vi "Get En and Ref Channels.vi"(11 "Reply Payload":T1 {"Settings"."EEG Channels"."16 EEG Channels"."Channel No" step=1}) -> (1 "Ch Names":string[](array[string]), 2 "Referenced Channels":u16, 3 "Enabled Channels":u16)   [LabVIEW 2016, in "Lab Streaming Layer.lvlib"]
uses:
  Lab Streaming Layer.lvlib
  Settings Editor/Update Application Settings (Reply Payload)--cluster.ctl
  Settings Editor/Settings--cluster.ctl
  Acquisition/Signal Type--enum.ctl
  Acquisition/Calibration Values--cluster.ctl
  CML Shared/EEG Channel Settings.ctl
  Acquisition/Acquisition.lvlib
  CML Shared/CML Shared.lvlib
  Settings Editor/Settings Editor.lvlib
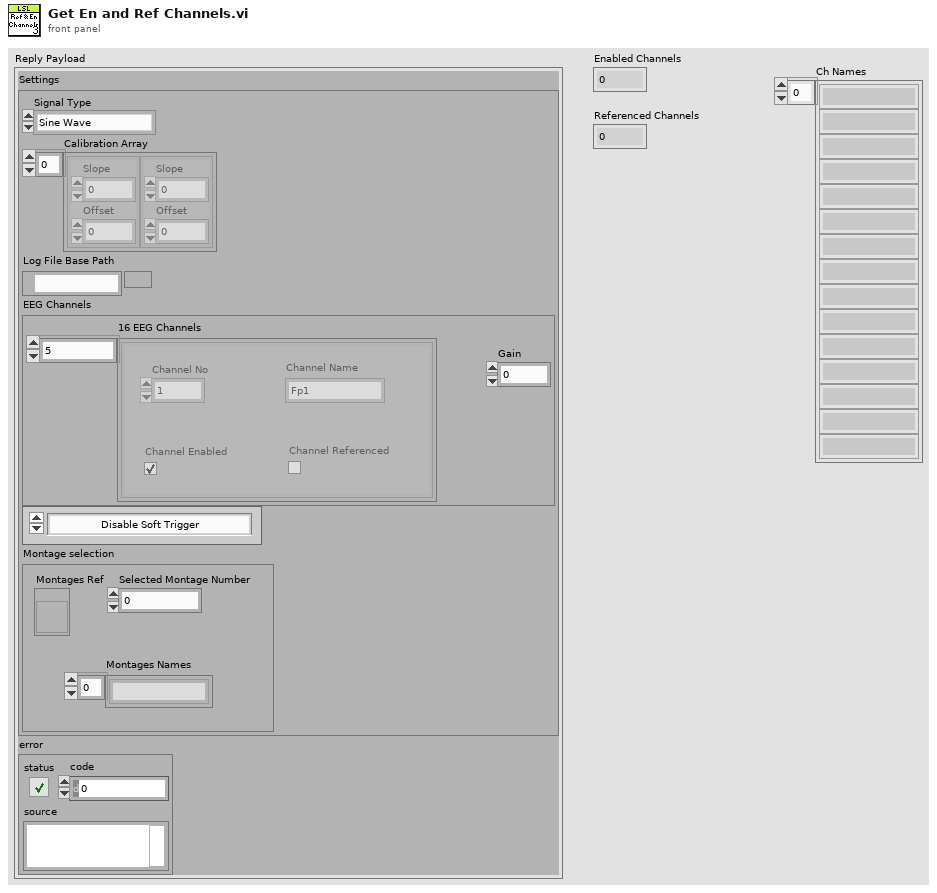
[diagram p1: front panel]
types:
  T1 = typedef "Settings Editor.lvlib/Update Application Settings (Reply Payload)--cluster.ctl" = cluster{"Settings":T2, "error":errorcluster}
  T2 = typedef "Settings Editor.lvlib/Settings--cluster.ctl" = cluster{"Signal Type":T3, "Calibration Array":T4[], "Log File Base Path":path, "EEG Channels":T5, "Soft Trig enum":enum16{"Disable Soft Trigger", "Enable Soft Trigger"}, "Montage selection":cluster{"Montages Ref":refnum<vi>, "Selected Montage Number":u8, "Montages Names":string[]}}
  T3 = typedef "Acquisition.lvlib/Signal Type--enum.ctl" = enum16{"Sine Wave", "Square with Noise"}
  T4 = typedef "Acquisition.lvlib/Calibration Values--cluster.ctl" = cluster{"Slope":dbl, "Offset":dbl}
  T5 = typedef "CML Shared.lvlib/EEG Channel Settings.ctl" = cluster{"16 EEG Channels":cluster{"Channel Name":string, "Channel No":u8, "Channel Enabled":bool, "Channel Referenced":bool}[], "Gain":u8}
  T6 = cluster{"Channel Name":string, "Channel No":u8, "Channel Enabled":bool, "Channel Referenced":bool}[]
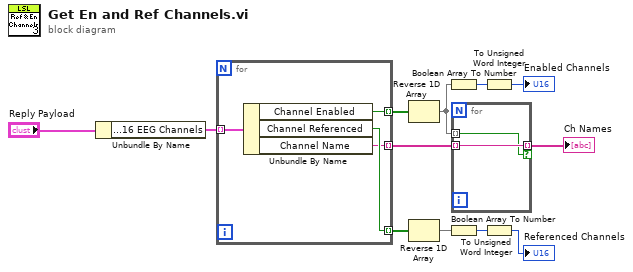
[diagram p0: block diagram]
diagram:
  n1 = Unbundle By Name("Reply Payload") -> ("Settings.EEG Channels.16 EEG Channels"=w7:T6)
  n2 = for {
    tunnel: w7 -> [w16] mode=indexing
    tunnel: [w15] -> w8 mode=indexing
    tunnel: [w14] -> w11 mode=indexing
    tunnel: [w13] -> w2 mode=indexing
    n3 = Unbundle By Name(w16) -> ("Channel Enabled"=w15:bool, "Channel Referenced"=w14:bool, "Channel Name"=w13:string)
  }
  n4 = Reverse 1D Array(array=w8) -> (reversed array=w3:bool[])
  n5 = Reverse 1D Array(array=w11) -> (reversed array=w12:bool[])
  n6 = Boolean Array To Number(Boolean array=w3) -> (number=w6:u32)
  n7 = Boolean Array To Number(Boolean array=w12) -> (number=w9:u32)
  n8 = for {
    tunnel: w3 -> [w17] mode=indexing
    tunnel: w2 -> [w18] mode=indexing
    tunnel: [w18] -> w1 mode=indexing if=w17
  }
  "Ch Names" <- w1
  n9 = To Unsigned Word Integer(number=w6) -> (unsigned 16bit integer=→"Enabled Channels":u16)
  n10 = To Unsigned Word Integer(number=w9) -> (unsigned 16bit integer=→"Referenced Channels":u16)
